vi "Calibration Complete.vi"(8 "error in":errorcluster, 11 "Calibration UI in":refnum<class "Calibration UI.lvclass">) -> (0 "error out":errorcluster, 3 "Calibration UI out":refnum<class "Calibration UI.lvclass">)   [LabVIEW 2015, in "Calibration UI.lvclass"]
uses:
  Calibration UI.lvclass
  Calibration UI.lvclass/Calibration UI.ctl
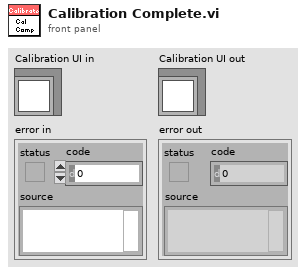
[diagram p1: front panel]
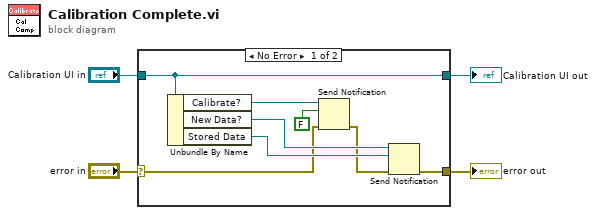
[diagram p0: block diagram]
diagram:
  n1 = case shown="No Error" "error in" {
    selector: "error in" -> [w6 w14]
    tunnel: [w5 w14] -> w3
    tunnel: [w11 w13] -> w1
    tunnel: "Calibration UI in" -> [w11 w13]
    frame No Error {
      n2 = Unbundle By Name(w11) -> ("Calibrate?"=w10:refnum<notifier>, "New Data?"=w8:refnum<notifier>, "Stored Data"=w9:refnum<data-value>)
      n3 = Send Notification(notification=FALSE, notifier=w10, error in (no error)=w6) -> (error out=w7:errorcluster)  [unwired: 1 out]
      n4 = Send Notification(notification=w9, notifier=w8, error in (no error)=w7) -> (error out=w5:errorcluster)  [unwired: 1 out]
    }
    frame Error {
    }
  }
  "error out" <- w3
  "Calibration UI out" <- w1
